vi "RotateAngle.vi"(6 "Reset?":bool=TRUE, 9 "RobotDriveDevRef":T1={"DevStatus"={"status"=FALSE, "code"=0, "source"=""}, "Motors[]"=[], "Square Inputs"=FALSE, "Max Output"=1.0, "Isochronous"=FALSE}, 10 "GyroDevRef":T9, 11 "Target":dbl format="%#_13g") -> (1 "RobotDriveDevRef 2":T1={"DevStatus"={"status"=FALSE, "code"=0, "source"=""}, "Motors[]"=[], "Square Inputs"=FALSE, "Max Output"=1.0, "Isochronous"=FALSE}, 2 "GyroDevRef 2":T9)   [LabVIEW 2013]
uses:
  <vilib>/Rock Robotics/WPI/Gyro/WPI_GyroDevRef.ctl
  <vilib>/Rock Robotics/SystemInterfaces/Typedef/FPGA_TypedefAnalogModule.ctl
  <vilib>/Rock Robotics/SystemInterfaces/AI/FPGA_AIChannel.ctl
  <vilib>/Rock Robotics/WPI/RobotDrive/WPI_RobotDriveDevRef.ctl
  <vilib>/Rock Robotics/WPI/MotorControl/WPI_MotorControlDeviceRef.ctl
  <vilib>/Rock Robotics/SystemInterfaces/Typedef/FPGA_TypedefDigitalModule.ctl
  <vilib>/Rock Robotics/SystemInterfaces/DIO/FPGA_DIOPWMChannel.ctl
  <vilib>/Rock Robotics/WPI/PWM/WPI_PWMDeadband.ctl
  <vilib>/Rock Robotics/WPI/CAN/Jaguar/SubVIs/WPI_CANJaguar_ControlMode.ctl
  <vilib>/Rock Robotics/WPI/PWM/WPI_PWMTransform_ConPane.ctl
  <vilib>/addons/control/pid/pid.llb/PID (DBL).vi
  <vilib>/addons/control/pid/NI_PID_pid.lvlib
panel:
  out "Array":dbl[](array[numeric])
  in  "output range 2":cluster{"output high":dbl, "output low":dbl}={"output high"=0.65, "output low"=-0.65}
  in  "PID gains 2":T12={"proportional gain (Kc)"=0.085, "integral time (Ti, min)"=0.0085, "derivative time (Td, min)"=0.0008}
  # "Stop?"
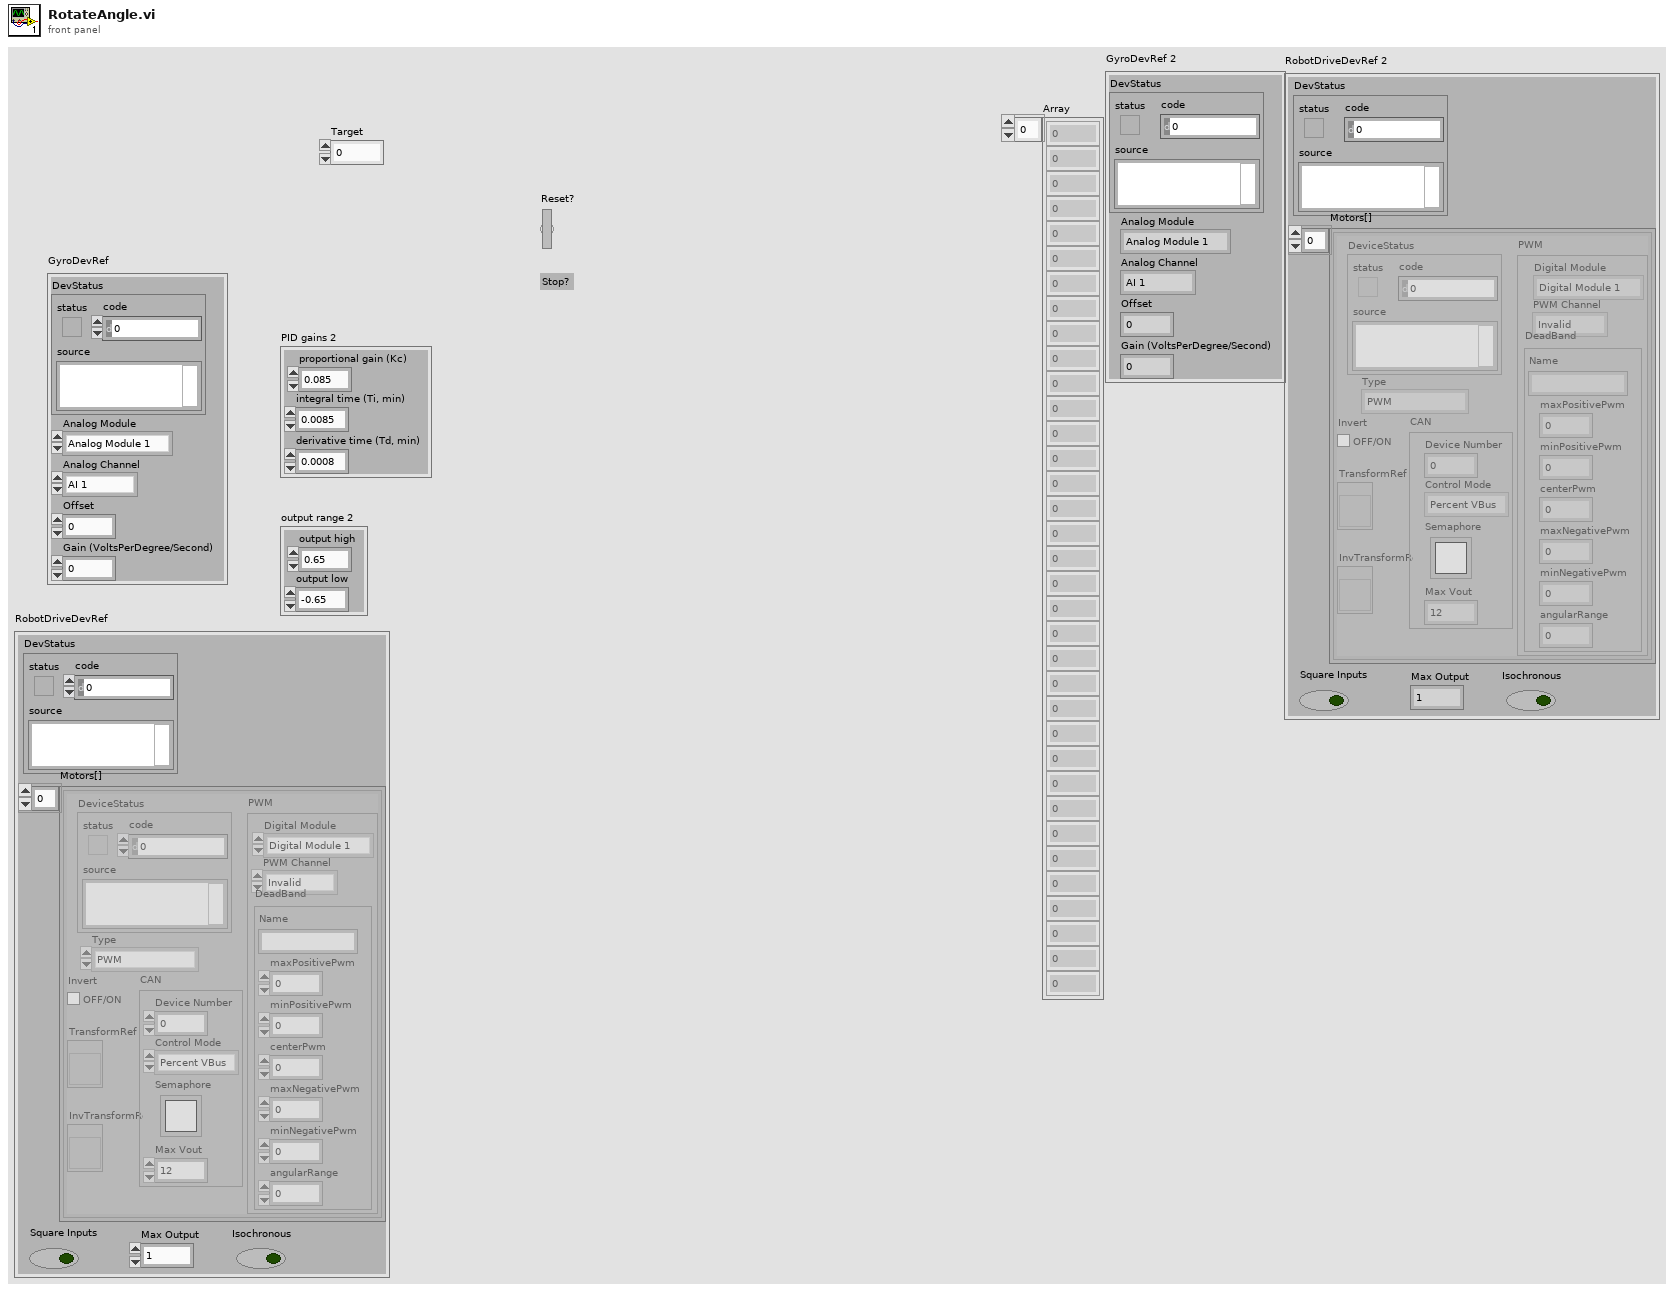
[diagram p1: front panel]
types:
  T1 = typedef "WPI_RobotDriveDevRef.ctl" = cluster{"DevStatus":errorcluster, "Motors[]":T2[], "Square Inputs":bool, "Max Output":dbl, "Isochronous":bool}
  T2 = typedef "WPI_MotorControlDeviceRef.ctl" = cluster{"DeviceStatus":errorcluster, "Type":enum16{"PWM", "CAN"}, "PWM":cluster{"Digital Module":T3, "PWM Channel":T4, "DeadBand":T5}, "CAN":cluster{"Device Number":u8, "Control Mode":T6, "Semaphore":T7, "Max Vout":dbl}, "Invert":bool, "TransformRef":T8, "InvTransformRef":T8}
  T3 = typedef "FPGA_TypedefDigitalModule.ctl" = enum16{"Digital Module 1", "Digital Module 2"}
  T4 = typedef "FPGA_DIOPWMChannel.ctl" = enum8{"PWM 1", "PWM 2", "PWM 3", "PWM 4", "PWM 5", "PWM 6", "PWM 7", "PWM 8", "PWM 9", "PWM 10", "Invalid"}
  T5 = typedef "WPI_PWMDeadband.ctl" = cluster{"Name":string, "maxPositivePwm":i32, "minPositivePwm":i32, "centerPwm":i32, "maxNegativePwm":i32, "minNegativePwm":i32, "angularRange":u16}
  T6 = typedef "WPI_CANJaguar_ControlMode.ctl" = enum8{"Percent VBus", "Current", "Speed", "Position", "Voltage"}
  T7 = typedef "Semaphore RefNum" = refnum<k1>
  T8 = typedef "WPI_PWMTransform_ConPane.ctl" = refnum<vi>
  T9 = typedef "WPI_GyroDevRef.ctl" = cluster{"DevStatus":errorcluster, "Analog Module":T10, "Analog Channel":T11, "Offset":dbl, "Gain (VoltsPerDegree/Second)":dbl}
  T10 = typedef "FPGA_TypedefAnalogModule.ctl" = enum16{"Analog Module 1", "Analog Module 2"}
  T11 = typedef "FPGA_AIChannel.ctl" = enum8{"AI 1", "AI 2", "AI 3", "AI 4", "AI 5", "AI 6", "AI 7", "AI 8", "Invalid"}
  T12 = cluster{"proportional gain (Kc)":dbl, "integral time (Ti, min)":dbl, "derivative time (Td, min)":dbl}
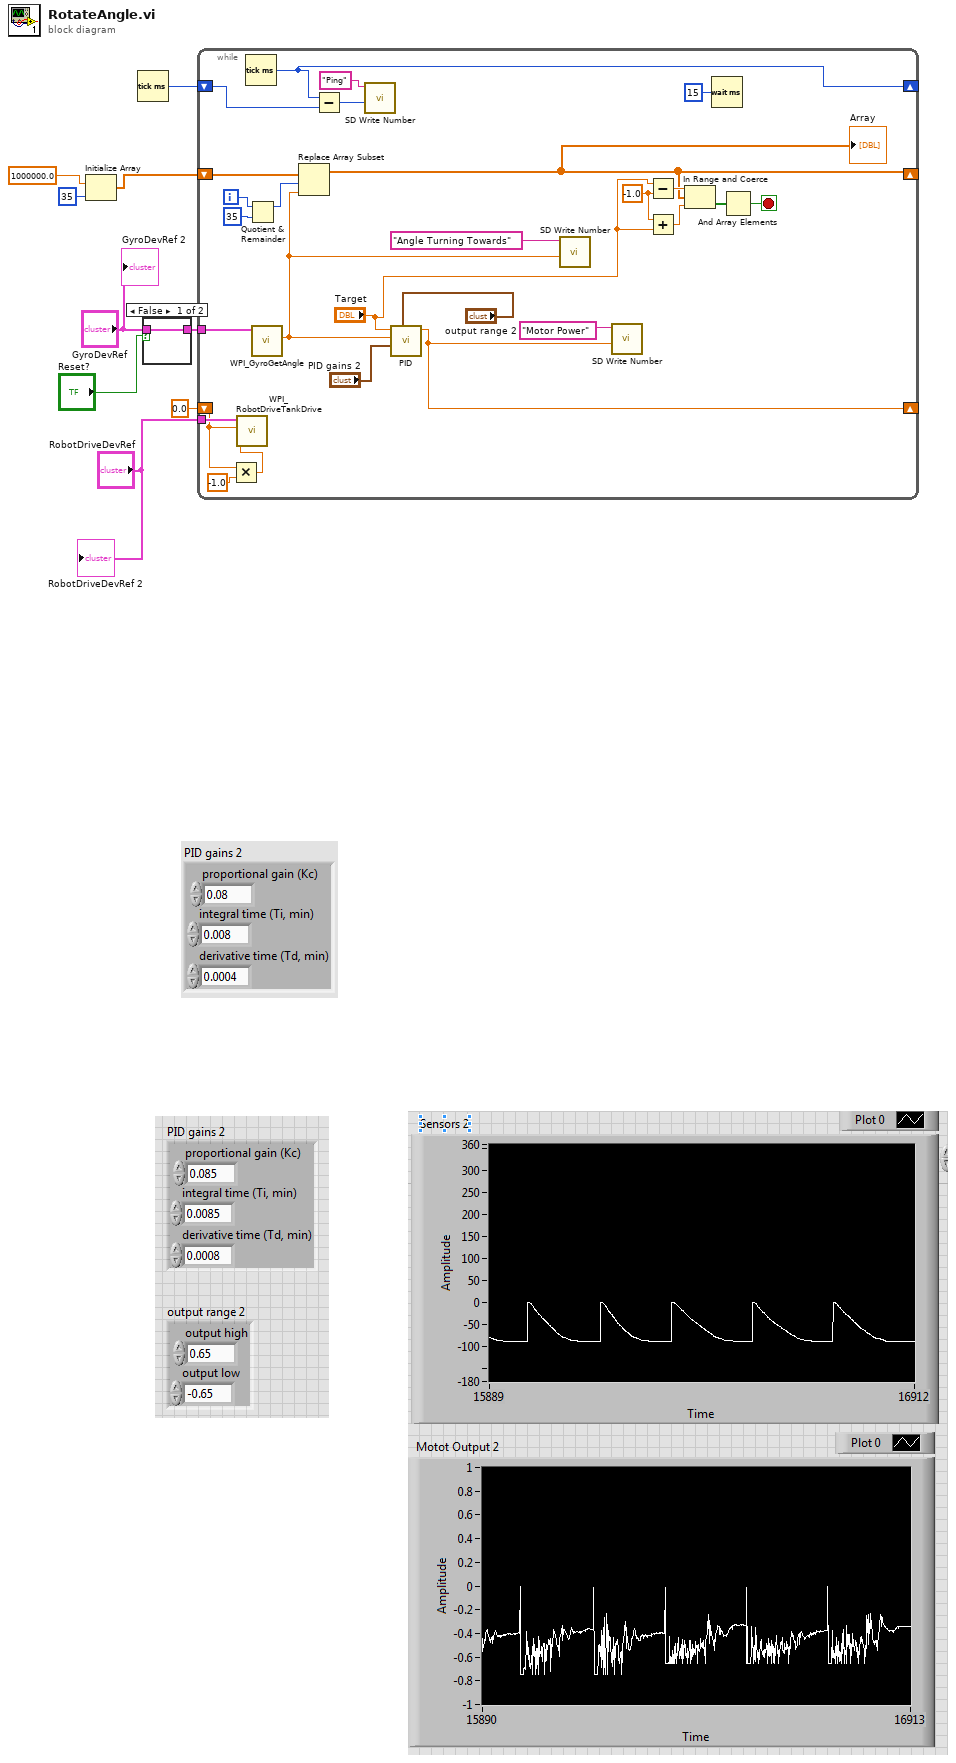
[diagram p0: block diagram]
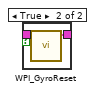
[diagram p2: hidden frame]
diagram:
  n1 = Initialize Array(1000000.0 ("element"), 35 ("dimension size")) -> (w3:dbl[])
  n2 = Tick Count (ms)() -> (millisecond timer value=w7:u32)
  n3 = case shown="False" "Reset?" {
    tunnel: [w10 w12] -> w9
    tunnel: "GyroDevRef" -> [w10 w11]
    frame False {
    }
    frame True {
      n4 = call <vilib>:"WPI_GyroReset.vi"("GyroDevRef"=w11) -> ("GyroDevRef"=w12:T9)  [unwired: 9 in, 1 out]
    }
  }
  n5 = while {
    tunnel: w9 -> [w18]
    shift-right: [w36] -> _
    shift-left: w7 -> [w37]
    shift-right: [w22] -> _
    shift-left: 0.0 ("output") -> [w31]
    tunnel: "RobotDriveDevRef" -> [w33]
    shift-right: [w16] -> _
    shift-left: w3 -> [w28]
    i -> [w20]
    stop <- w26 stop-if-true
    w14 = -1.0 ("y")
    n6 = Multiply(x=w31, y=-1.0) -> (x*y=w35:dbl)
    n7 = call <vilib>:"WPI_RobotDriveTankDrive.vi"("Right axis value"=w35, "Left axis value"=w31, "RobotDriveDevRef"=w33) -> ()  [unwired: 6 in, 3 out]
    n8 = Tick Count (ms)() -> (millisecond timer value=w36:u32)
    n9 = Quotient & Remainder(x=w20, y=35) -> (x-y*floor(x/y)=w29:i32)  [unwired: 1 out]
    n10 = call <vilib>:"WPI_GyroGetAngle.vi"("GyroDevRef"=w18) -> ("Angle"=w19:dbl)  [unwired: 7 in, 3 out]
    n11 = Replace Array Subset(array=w28, new element=w19, index=w29) -> (w16:dbl[])
    "Array" <- w16
    n12 = Subtract(x=w36, y=w37) -> (x-y=w24:u32)
    n13 = call <vilib>:"SD Write Number.vi"("Numeric"=w24, "Name"="Ping") -> ()  [unwired: 8 in, 2 out]
    n14 = call-poly <vilib>:"PID.vi"("output range"="output range 2", "PID gains"="PID gains 2", "process variable"=w19, "setpoint"="Target") -> ("output"=w22:dbl)  [unwired: 6 in, 1 out]
    n15 = call <vilib>:"SD Write Number.vi"("Numeric"=w19, "Name"="Angle Turning Towards") -> ()  [unwired: 8 in, 2 out]
    n16 = call <vilib>:"SD Write Number.vi"("Numeric"=w22, "Name"="Motor Power") -> ()  [unwired: 8 in, 2 out]
    n17 = Subtract(x="Target", y=w14) -> (x-y=w27:dbl)
    n18 = Add(x=w14, y="Target") -> (x+y=w15:dbl)
    n19 = In Range and Coerce(upper limit=w27, x=w16, lower limit=w15) -> (In Range?=w17:bool[])  [unwired: 1 out]
    n20 = Wait (ms)(milliseconds to wait=u32 15) -> ()  [unwired: 1 out]
    n21 = And Array Elements(Boolean array=w17) -> (logical AND=w26:bool)
  }
  "GyroDevRef 2" <- "GyroDevRef"
  "RobotDriveDevRef 2" <- "RobotDriveDevRef"
